vi "request.vi"(0 "URL":string, 1 "headers":string[](array[string]), 2 "POST Payload":string, 3 "error in":errorcluster, 4 "method":string="get") -> (8 "Comm":T1, 10 "error out":errorcluster)   [LabVIEW 2022 SP3]
uses:
  HTTPComm.ctl
  <vilib>/httpClient/POSTBuffer.vi
  <vilib>/httpClient/LabVIEWHTTPClient.lvlib
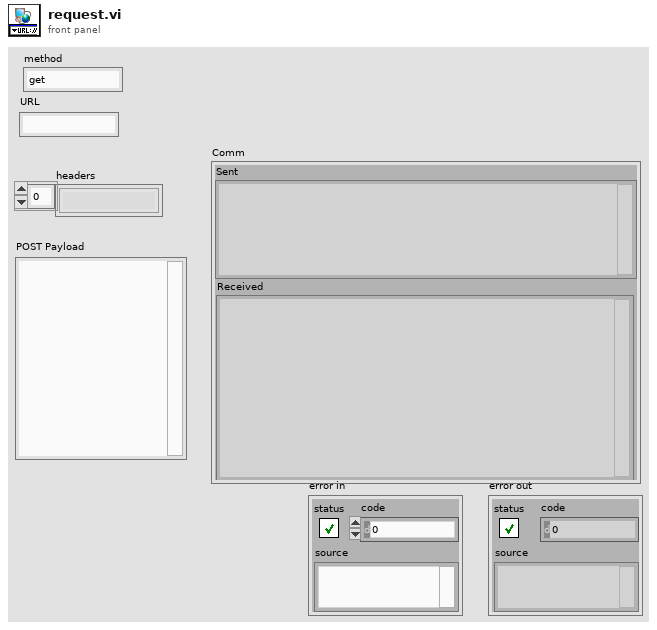
[diagram p1: front panel]
types:
  T1 = typedef "HTTPComm.ctl" = cluster{"url":string, "sent headers":string, "sent body":string, "headers":string, "body":string, "Sent":string, "Received":string}
  T2 = typedef "LabVIEWHTTPClient.lvlib/ClientHandle.ctl" = refnum<k1>
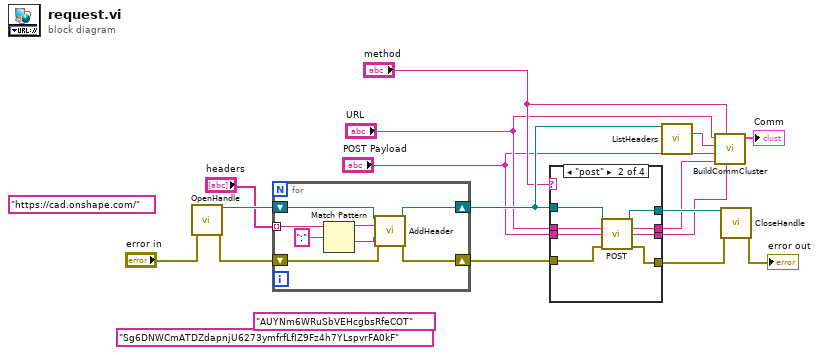
[diagram p0: block diagram]
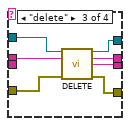
[diagram p3: hidden frame]
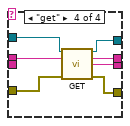
[diagram p4: hidden frame]
diagram:
  (unwired) "https://cad.onshape.com/" ("method")
  (unwired) "Sg6DNWCmATDZdapnjU6273ymfrfLfIZ9Fz4h7YLspvrFA0kF" ("password")
  (unwired) "AUYNm6WRuSbVEHcgbsRfeCOT" ("username")
  n1 = call <vilib>:"OpenHandle.vi"("error in (no error)"="error in") -> ("client handle out"=w15:T2, "error out"=w13:errorcluster)  [unwired: 13 in]
  n2 = for {
    shift-right: [w23] -> w10
    shift-left: w15 -> [w24]
    shift-right: [w21] -> w12
    shift-left: w13 -> [w22]
    tunnel: "headers" -> [w17] mode=indexing
    n3 = Match Pattern(string=w17, regular expression=":") -> (before substring=w19:string, after substring=w18:string)  [unwired: 1 in, 2 out]
    n4 = call <vilib>:"AddHeader.vi"("client handle"=w24, "header"=w19, "value"=w18, "error in (no error)"=w22) -> ("client handle out"=w23:T2, "error out"=w21:errorcluster)  [unwired: 10 in]
  }
  n5 = case shown="\"post\"" "method" {
    tunnel: w10 -> [_ w33 w40 w47]
    tunnel: [_ w26 w39 w46] -> w16
    tunnel: [_ w32 w37 w44] -> w7
    tunnel: [_ w31 w38 w45] -> w8
    tunnel: w12 -> [w25 w30 w36 w43]
    tunnel: [w25 w29 w35 w42] -> w5
    tunnel: "URL" -> [_ w28 w34 w41]
    tunnel: "POST Payload" -> [_ w27 _ _]
    frame Default {
    }
    frame "post" {
      n6 = call-poly <vilib>:"POST.vi"("client handle"=w33, "url"=w28, "buffer"=w27, "error in (no error)"=w30) -> ("client handle out"=w26:T2, "headers"=w31:string, "body"=w32:string, "error out"=w29:errorcluster)  [unwired: 8 in]
    }
    frame "delete" {
      n7 = call <vilib>:"DELETE.vi"("client handle"=w40, "url"=w34, "error in (no error)"=w36) -> ("client handle out"=w39:T2, "headers"=w38:string, "body"=w37:string, "error out"=w35:errorcluster)  [unwired: 9 in]
    }
    frame "get" {
      n8 = call <vilib>:"GET.vi"("client handle"=w47, "url"=w41, "error in (no error)"=w43) -> ("client handle out"=w46:T2, "headers"=w45:string, "body"=w44:string, "error out"=w42:errorcluster)  [unwired: 9 in]
    }
  }
  n9 = call <vilib>:"ListHeaders.vi"("client handle"=w10) -> ("headers"=w9:string)  [unwired: 12 in, 2 out]
  n10 = call "BuildCommCluster.vi"("reply body"=w7, "Type"="method", "reply headers"=w8, "sent body"="POST Payload", "sent headers"=w9, "url"="URL") -> ("Comm"=→"Comm":T1)  [unwired: 5 in]
  n11 = call <vilib>:"CloseHandle.vi"("client handle"=w16, "error in (no error)"=w5) -> ("error out"=→"error out":errorcluster)  [unwired: 13 in]
